vi "Right Click Menu Activated.vi"(8 "error in (no error)":errorcluster, 10 "MenuRef":refnum<k9>, 11 "SubPanel User Interface in":refnum<class "SubPanel User Interface.lvclass">) -> (0 "error out":errorcluster, 3 "SubPanel User Interface out":refnum<class "SubPanel User Interface.lvclass">)   [LabVIEW 2020, in "SubPanel User Interface.lvlib" / "SubPanel User Interface.lvclass"]
uses:
  SubPanel User Interface.lvclass
  SubPanel User Interface.lvclass/SubPanel User Interface.ctl
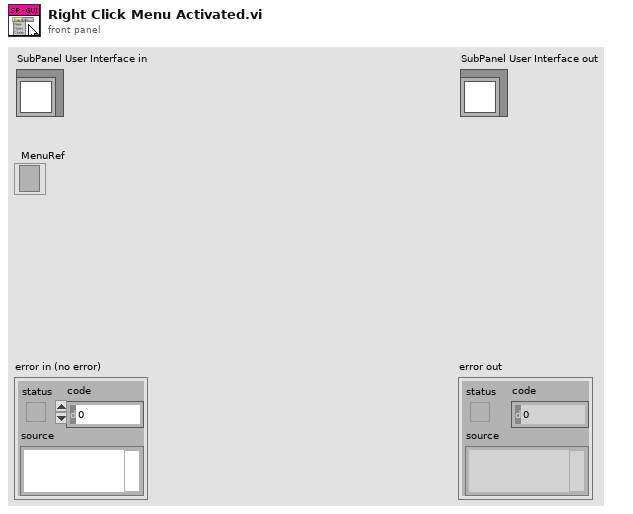
[diagram p1: front panel]
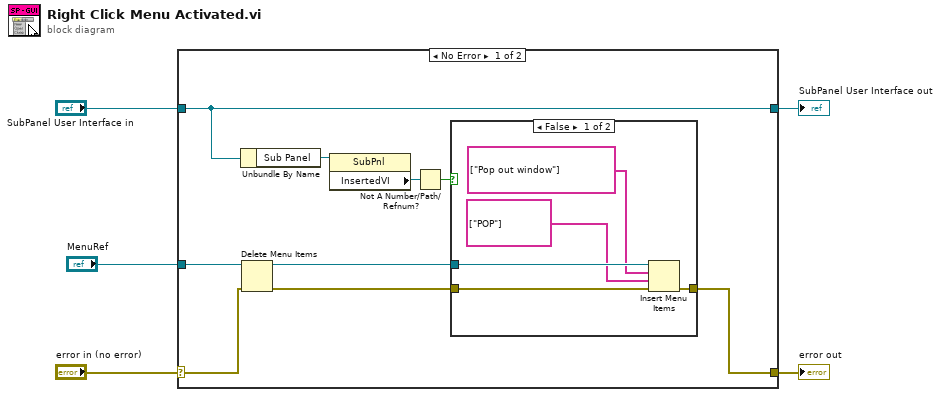
[diagram p0: block diagram]
diagram:
  n1 = case shown="No Error" "error in (no error)" {
    selector: "error in (no error)" -> [w7 w22]
    tunnel: [w6 w22] -> w4
    tunnel: [w14 w21] -> w2
    tunnel: "SubPanel User Interface in" -> [w14 w21]
    tunnel: "MenuRef" -> [w10 _]
    frame No Error {
      n2 = Unbundle By Name(w14) -> ("Sub Panel"=w13:refnum<vi>)
      n3 = Delete Menu Items(6:w7, 9:w10) -> (0:w8:errorcluster, 3:w9:refnum<k9>)  [unwired: 2 in]
      n4 = property class="SubPnl"(reference=w13) -> ("InsertedVI"=w12:refnum<vi>)  [unwired: 1 in, 2 out]
      n5 = Not A Number/Path/Refnum?(number/path/refnum=w12) -> (NaN/Path/Refnum?=w11:bool)
      n6 = case shown="False" w11 {
        tunnel: w9 -> [w19 _]
        tunnel: w8 -> [w18 w20]
        tunnel: [w17 w20] -> w6
        frame False {
          n7 = Insert Menu Items(6:w18, 7:string[] ["POP"] ("item tags"), 8:string[] ["Pop out window"], 9:w19) -> (0:w17:errorcluster)  [unwired: 2 in, 2 out]
        }
        frame True {
        }
      }
    }
    frame Error {
    }
  }
  "error out" <- w4
  "SubPanel User Interface out" <- w2
